vi "Write Rate (Hz).vi"(8 "error in (no error)":errorcluster, 10 "Rate (Hz)":dbl, 11 "Change Laser Rep Rate in":refnum<class "Change Laser Rep Rate.lvclass">) -> (0 "error out":errorcluster, 3 "Change Laser Rep Rate out":refnum<class "Change Laser Rep Rate.lvclass">)   [LabVIEW 2014, in "eCRDS Library.lvlib" / "Change Laser Rep Rate.lvclass"]
uses:
  Change Laser Rep Rate.lvclass
  Change Laser Rep Rate.lvclass/Change Laser Rep Rate.ctl
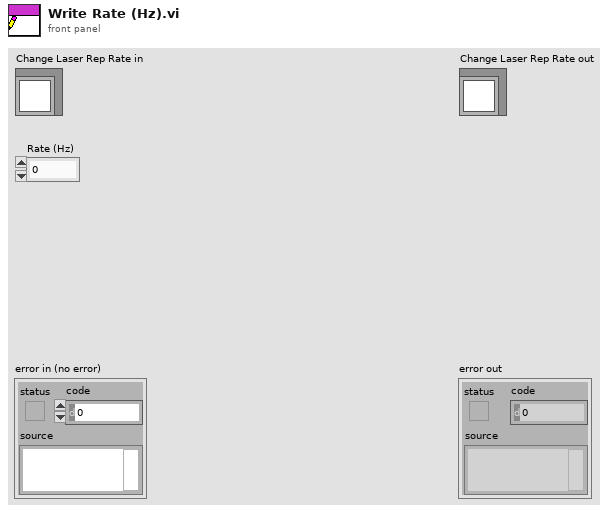
[diagram p1: front panel]
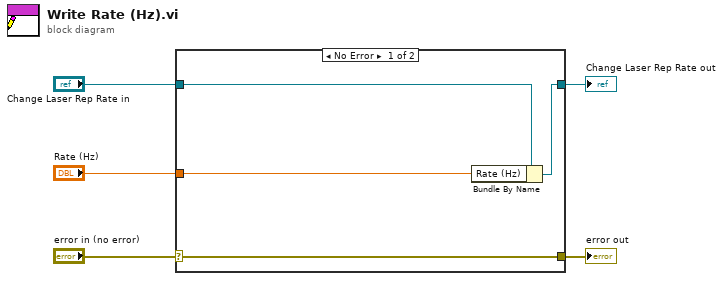
[diagram p0: block diagram]
diagram:
  n1 = case shown="No Error" "error in (no error)" {
    selector: "error in (no error)" -> [w9 w10]
    tunnel: [w9 w10] -> w4
    tunnel: [w7 w11] -> w2
    tunnel: "Change Laser Rep Rate in" -> [w8 w11]
    tunnel: "Rate (Hz)" -> [w6 _]
    frame No Error {
      n2 = Bundle By Name(cluster=w8, "Rate (Hz)"=w6) -> (w7:refnum<class "Change Laser Rep Rate.lvclass">)
    }
    frame Error {
    }
  }
  "error out" <- w4
  "Change Laser Rep Rate out" <- w2
